vi "TDMS - Perform DAQ Data.vi"(8 "error in (no error)":errorcluster, 10 "RT Data portion":dbl[](array[numeric]), 11 "View Model":T1) -> (0 "error out":errorcluster, 3 "View Model":T1)   [LabVIEW 2017]
doc: "This SubVI perform DAQ data from RT Data portion before saving to TDMS."
uses:
  View Model/Controls/View Model.ctl
  View Model/Controls/Shared Model.ctl
  Error Handler/Controls/Error Model.ctl
  Error Handler/Controls/Error Event.ctl
  Error Handler/Controls/Error Type.ctl
  Controller/Controls/Controller Model.ctl
  Controller/Controls/Controller Event.ctl
  Controller/Controls/Controller Command.ctl
  Controller/Controls/Controller Overhead.ctl
  Real-Time/RT Status.ctl
  Real-Time/RT Loop Status.ctl
  Controller/Controls/Controller NStream.ctl
  Controller/Controls/Controller Timer Data.ctl
  Controller/Controls/Controller DAQ Data.ctl
  Controls/TDMS Model.ctl
  Controls/TDMS Event.ctl
  Controls/TDMS Command.ctl
  Controls/TDMS Overhead.ctl
  Controls/TDMS ChanProperties.ctl
  Controls/TDMS DAQ Data.ctl
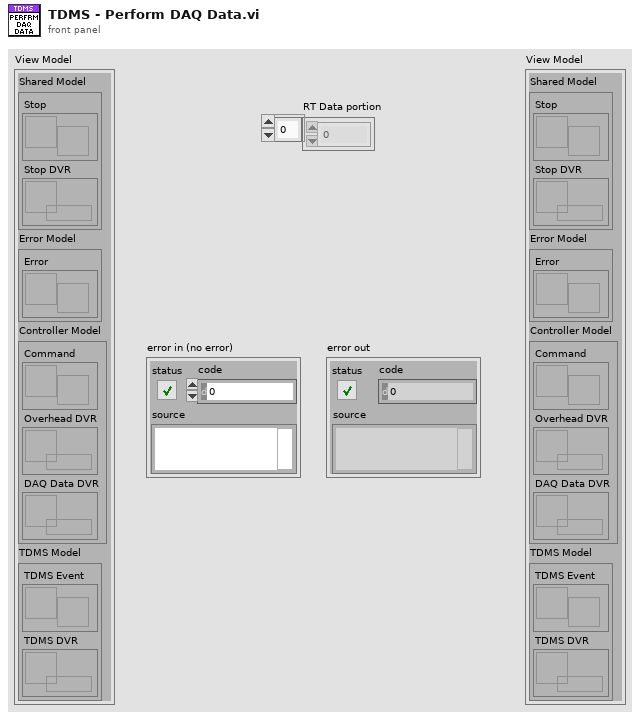
[diagram p1: front panel]
types:
  T1 = typedef "View Model.ctl" = cluster{"Shared Model":T2, "Error Model":T3, "Controller Model":T4, "TDMS Model":T5}
  T2 = typedef "Shared Model.ctl" = cluster{"Stop":refnum<user-event>, "Stop DVR":refnum<data-value>}
  T3 = typedef "Error Model.ctl" = cluster{"Error":refnum<user-event>}
  T4 = typedef "Controller Model.ctl" = cluster{"Command":refnum<user-event>, "Overhead DVR":refnum<data-value>, "DAQ Data DVR":refnum<data-value>}
  T5 = typedef "TDMS Model.ctl" = cluster{"TDMS Event":refnum<user-event>, "TDMS DVR":refnum<data-value>}
  T6 = typedef "TDMS DAQ Data.ctl" = cluster{"AOM data":dbl[], "AIMV data":dbl[], "AIMC data":dbl[], "DOM data":dbl[], "DIM data":dbl[], "AOM timestamp":dbl, "AIMV timestamp":dbl, "AIMC timestamp":dbl, "DOM timestamp":dbl, "DIM timestamp":dbl}
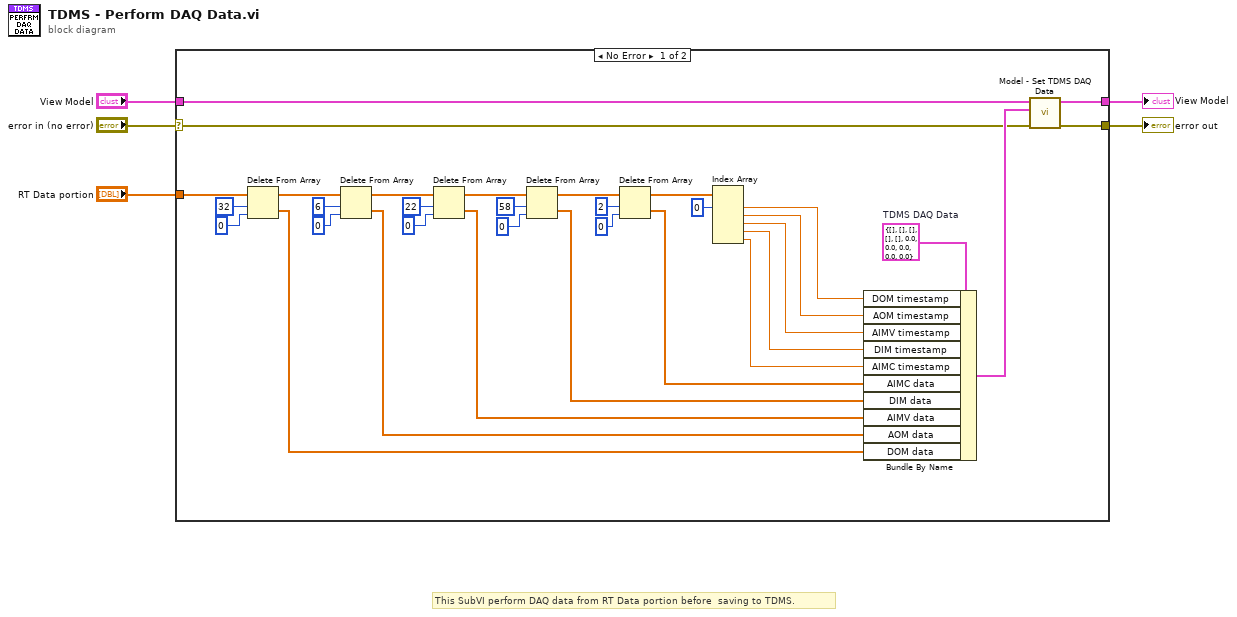
[diagram p0: block diagram]
diagram:
  # "This SubVI perform DAQ data from RT Data portion before  saving to TDMS."
  n1 = case shown="No Error" "error in (no error)" {
    selector: "error in (no error)" -> [w7 w39]
    tunnel: [w6 w39] -> w4
    tunnel: "View Model" -> [w10 w40]
    tunnel: [w9 w40] -> w2
    tunnel: "RT Data portion" -> [w12 _]
    frame No Error {
      w11 = T6 {"AOM data"=[], "AIMV data"=[], "AIMC data"=[], "DOM data"=[], "DIM data"=[], "AOM timestamp"=0.0, "AIMV timestamp"=0.0, "AIMC timestamp"=0.0, "DOM timestamp"=0.0, "DIM timestamp"=0.0}  # TDMS DAQ Data
      n2 = Delete From Array(array=w12, length=32, index=0) -> (deleted portion=w36:dbl[], array with subset deleted=w35:dbl[])
      n3 = Delete From Array(array=w35, length=6, index=0) -> (deleted portion=w32:dbl[], array with subset deleted=w31:dbl[])
      n4 = Delete From Array(array=w31, length=22, index=0) -> (deleted portion=w28:dbl[], array with subset deleted=w25:dbl[])
      n5 = Delete From Array(array=w25, length=58, index=0) -> (deleted portion=w24:dbl[], array with subset deleted=w21:dbl[])
      n6 = Delete From Array(array=w21, length=2, index=0) -> (deleted portion=w20:dbl[], array with subset deleted=w13:dbl[])
      n7 = Index Array(array=w13, index #1=0 ("index")) -> (element #1=w14:dbl, element #2=w15:dbl, element #3=w16:dbl, element #4=w17:dbl, element #5=w18:dbl)  [unwired: 4 in]
      n8 = Bundle By Name(cluster=w11, "DOM timestamp"=w14, "AOM timestamp"=w15, "AIMV timestamp"=w16, "DIM timestamp"=w17, "AIMC timestamp"=w18, "AIMC data"=w20, "DIM data"=w24, "AIMV data"=w28, "AOM data"=w32, "DOM data"=w36) -> (w8:T6)
      n9 = call "Model - Set TDMS DAQ Data.vi"("error in (no error)"=w7, "TDMS DAQ Data"=w8, "View Model"=w10) -> ("error out"=w6:errorcluster, "View Model"=w9:T1)  [unwired: 7 in]
    }
    frame Error {
    }
  }
  "View Model" <- w2
  "error out" <- w4
